vi "setUp.vi"(8 "error in (no error)":errorcluster, 11 "reference in":refnum<class "BufferedArray_Functional.lvclass">) -> (0 "error out":errorcluster, 3 "reference in":refnum<class "BufferedArray_Functional.lvclass">)   [LabVIEW 2009, in "BufferedArray_Functional.lvclass"]
doc: "setUp runs prior to the test method during test execution. Use this method to initialize any object data required by your tests."
uses:
  BufferedArray_Functional.lvclass
  source/Lists.Implementations/BufferedArray/BufferedArray.lvclass
  BufferedArray_Functional.lvclass/BufferedArray_Functional.ctl
  <vilib>/addons/_JKI Toolkits/VI Tester/TestCase.llb/TestCase.lvclass
  source/Lists/List/List.lvclass
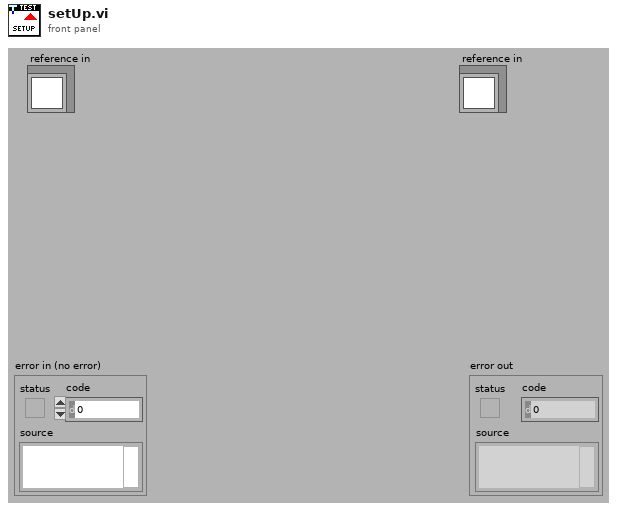
[diagram p1: front panel]
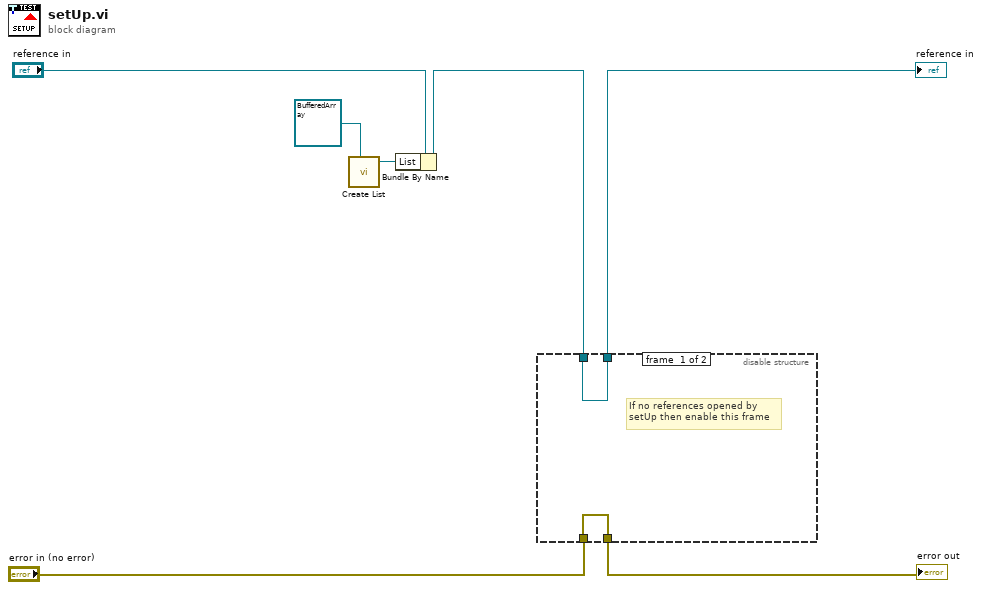
[diagram p0: block diagram]
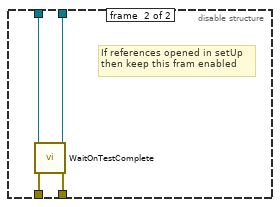
[diagram p2: hidden frame]
diagram:
  n1 = call "Create List.vi"("List Implementation (Array)"=refnum<class "BufferedArray.lvclass"> refnum ("LapDog.Collections.v0.Lists.Implementations.lvlib:BufferedArray.lvclass")) -> ("List out"=w2:refnum<class "List.lvclass">)  [unwired: 9 in, 1 out]
  n2 = Bundle By Name(cluster="reference in", "List"=w2) -> (w3:refnum<class "BufferedArray_Functional.lvclass">)
  n3 = disable-structure shown="Enabled" {
    disable-tunnel: w3 -> [w9 w13]
    disable-tunnel: [w9 w12] -> w4
    disable-tunnel: "error in (no error)" -> [w8 w11]
    disable-tunnel: [w8 w10] -> w6
    frame #0 {
      # "If no references opened by\nsetUp then enable this frame"
    }
    frame #1 {
      # "If references opened in setUp\nthen keep this fram enabled"
      n4 = call <vilib>:"WaitOnTestComplete.vi"("error in (no error)"=w11, "TestCase in"=w13) -> ("error out"=w10:errorcluster, "TestCase out"=w12:refnum<class "BufferedArray_Functional.lvclass">)  [unwired: 8 in]
    }
  }
  "error out" <- w6
  "reference in" <- w4
